vi "EjerciciodeWhile_Tanque.vi"() -> ()   [LabVIEW 2022 SP3]
panel:
  out "Terminado":bool
  out "Llenando":bool
  out "Tank":dbl(slide) scale=0.0..10.0
  in  "stop":bool
  # "Llenado de Tanque"
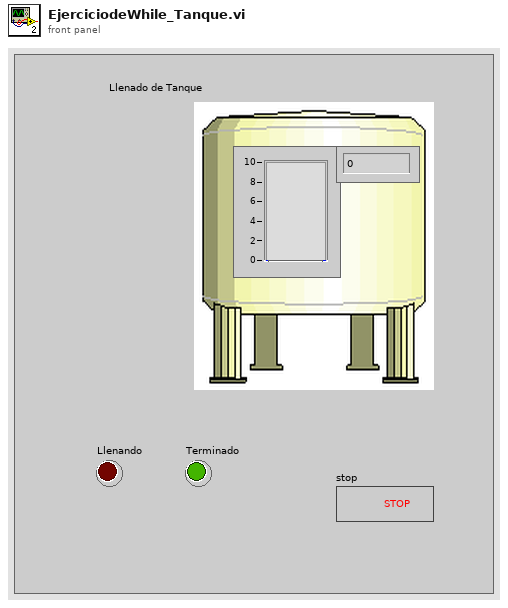
[diagram p1: front panel]
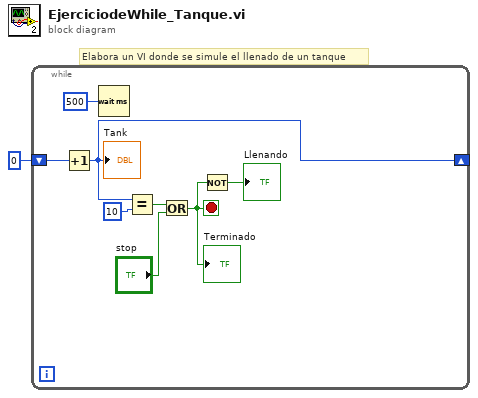
[diagram p0: block diagram]
diagram:
  # "Elabora un VI donde se simule el llenado de un tanque"
  n1 = while {
    shift-right: [w7] -> _
    shift-left: 0 -> [w9]
    stop <- w3 stop-if-true
    n2 = Increment(x=w9) -> (x+1=w7:i32)
    "Tank" <- w7
    n3 = Wait (ms)(milliseconds to wait=u32 500) -> ()  [unwired: 1 out]
    n4 = Equal?(x=w7, y=10) -> (x = y?=w5:bool)
    n5 = Or(x=w5, y="stop") -> (x .or. y?=w3:bool)
    "Terminado" <- w3
    n6 = Not(x=w3) -> (.not. x?=→"Llenando":bool)
  }
